vi "Config.vi"(8 "error in":errorcluster, 10 "Sporks Number":i32, 11 "VISA resource in":refnum<visa-resource-name>) -> (0 "error out":errorcluster, 1 "No response":bool, 3 "VISA resource out":refnum<visa-resource-name>)   [LabVIEW 2025]
uses:
  <vilib>/Utility/error.llb/Trim Whitespace One-Sided.vi
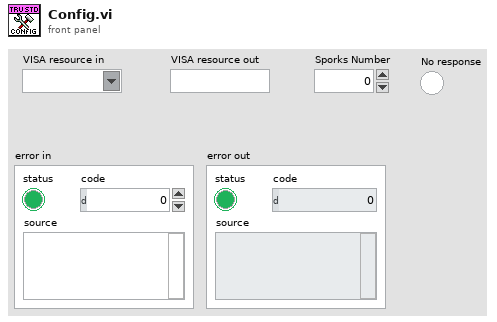
[diagram p1: front panel]
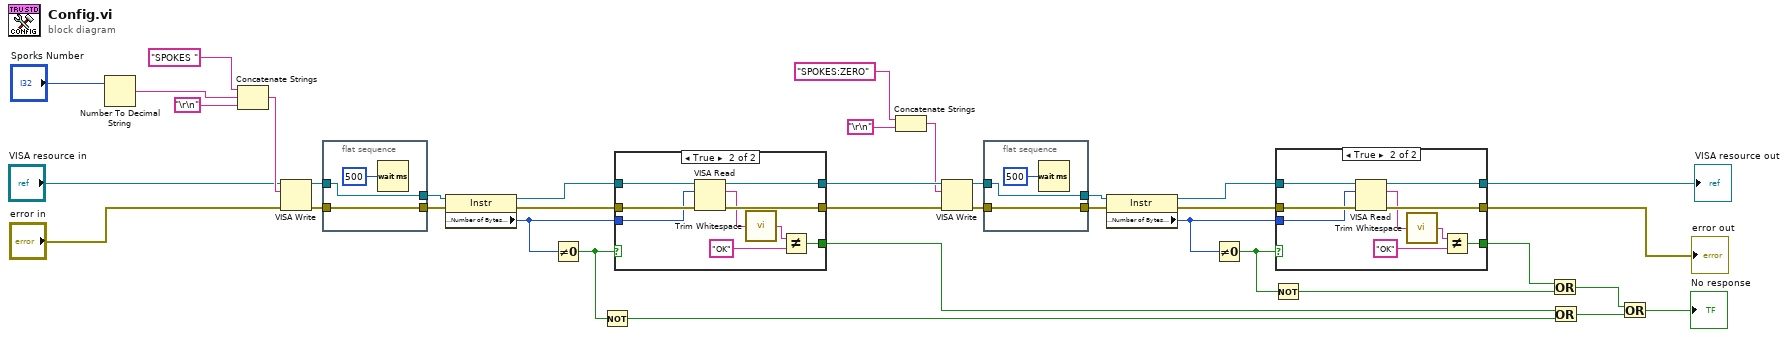
[diagram p0: block diagram]
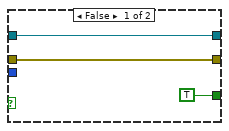
[diagram p2: hidden frame]
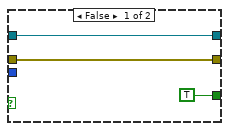
[diagram p3: hidden frame]
diagram:
  n1 = Number To Decimal String(number="Sporks Number") -> (decimal integer string=w31:string)  [unwired: 1 in]
  n2 = Concatenate Strings("SPOKES " ("string"), w31, "\r\n") -> (w36:string)
  n3 = VISA Write(VISA resource name="VISA resource in", write buffer=w36, error in (no error)="error in") -> (VISA resource name out=w32:refnum<visa-resource-name>, error out=w35:errorcluster)  [unwired: 1 out]
  n4 = flat-sequence {
    tunnel: [w39] -> w33
    tunnel: w32 -> [w39]
    tunnel: [w38] -> w34
    tunnel: w35 -> [w38]
    frame #0 {
      n5 = Wait (ms)(milliseconds to wait=u32 500) -> ()  [unwired: 1 out]
    }
  }
  n6 = property class="Instr"(reference=w33, error in=w34) -> (reference out=w27:refnum<visa-resource-name>, error out=w28:errorcluster, "Serial Settings:Number of Bytes at Serial Port"=w26:u32)
  n7 = Not Equal To 0?(x=w26) -> (x != 0?=w29:bool)
  n8 = Not(x=w29) -> (.not. x?=w24:bool)
  n9 = case shown="True" w29 {
    tunnel: w28 -> [w43 w52]
    tunnel: [w43 w51] -> w15
    tunnel: w27 -> [w42 w50]
    tunnel: [w42 w49] -> w16
    tunnel: w26 -> [_ w48]
    tunnel: [TRUE w44] -> w25
    frame False {
    }
    frame True {
      n10 = VISA Read(VISA resource name=w50, byte count=w48, error in (no error)=w52) -> (VISA resource name out=w49:refnum<visa-resource-name>, read buffer=w47:string, error out=w51:errorcluster)  [unwired: 1 out]
      n11 = call <vilib>:"Trim Whitespace.vi"("string"=w47) -> ("trimmed string"=w46:string)  [unwired: 1 in]
      n12 = Not Equal?(x=w46, y="OK") -> (x != y?=w44:bool)
    }
  }
  n13 = Concatenate Strings("SPOKES:ZERO" ("string"), "\r\n") -> (w7:string)
  n14 = VISA Write(VISA resource name=w16, write buffer=w7, error in (no error)=w15) -> (VISA resource name out=w20:refnum<visa-resource-name>, error out=w23:errorcluster)  [unwired: 1 out]
  n15 = flat-sequence {
    tunnel: [w54] -> w21
    tunnel: w20 -> [w54]
    tunnel: [w53] -> w22
    tunnel: w23 -> [w53]
    frame #0 {
      n16 = Wait (ms)(milliseconds to wait=u32 500) -> ()  [unwired: 1 out]
    }
  }
  n17 = property class="Instr"(reference=w21, error in=w22) -> (reference out=w18:refnum<visa-resource-name>, error out=w19:errorcluster, "Serial Settings:Number of Bytes at Serial Port"=w17:u32)
  n18 = Not Equal To 0?(x=w17) -> (x != 0?=w2:bool)
  n19 = Not(x=w2) -> (.not. x?=w3:bool)
  n20 = case shown="True" w2 {
    tunnel: w19 -> [w58 w67]
    tunnel: [w58 w66] -> w14
    tunnel: w18 -> [w57 w65]
    tunnel: [w57 w64] -> w13
    tunnel: w17 -> [_ w63]
    tunnel: [TRUE w59] -> w12
    frame False {
    }
    frame True {
      n21 = VISA Read(VISA resource name=w65, byte count=w63, error in (no error)=w67) -> (VISA resource name out=w64:refnum<visa-resource-name>, read buffer=w62:string, error out=w66:errorcluster)  [unwired: 1 out]
      n22 = call <vilib>:"Trim Whitespace.vi"("string"=w62) -> ("trimmed string"=w61:string)  [unwired: 1 in]
      n23 = Not Equal?(x=w61, y="OK") -> (x != y?=w59:bool)
    }
  }
  "VISA resource out" <- w13
  "error out" <- w14
  n24 = Or(x=w12, y=w3) -> (x .or. y?=w9:bool)
  n25 = Or(x=w25, y=w24) -> (x .or. y?=w10:bool)
  n26 = Or(x=w9, y=w10) -> (x .or. y?=→"No response":bool)
